vi "EnableControl.vi"(0 "Enable":bool, 1 "Reference":refnum<vi>) -> ()   [LabVIEW 2009]
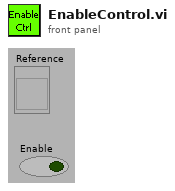
[diagram p1: front panel]
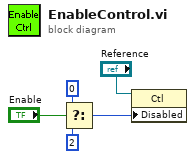
[diagram p0: block diagram]
diagram:
  n1 = Select(t=u8 0 ("Disabled"), s="Enable", f=u8 2 ("Disabled")) -> (s? t:f=w5:u8)
  n2 = property class="Ctl"(reference="Reference", "Disabled"=w5) -> ()  [unwired: 1 in, 2 out]
